vi "PostImagesONE_GRAPH_WORKING_PRE_LOOPIFY.vi"(6 "URL":string, 7 "Experiment Identifier":string, 8 "Transconductance..":refnum<vi>, 9 "Transconductance":refnum<vi>, 10 "Conductance..":refnum<vi>, 11 "Conductance":refnum<vi>) -> ()   [LabVIEW 2016]
uses:
  <vilib>/httpClient/MultipartData.ctl
  <vilib>/httpClient/POSTFile.vi
  <vilib>/httpClient/LabVIEWHTTPClient.lvlib
panel:
  out "error out 4":errorcluster
  out "error out 3":errorcluster
  out "error out 2":errorcluster
  out "error out":errorcluster
  out "appended path 4":path
  out "appended path 3":path
  out "appended path 2":path
  out "appended path":path
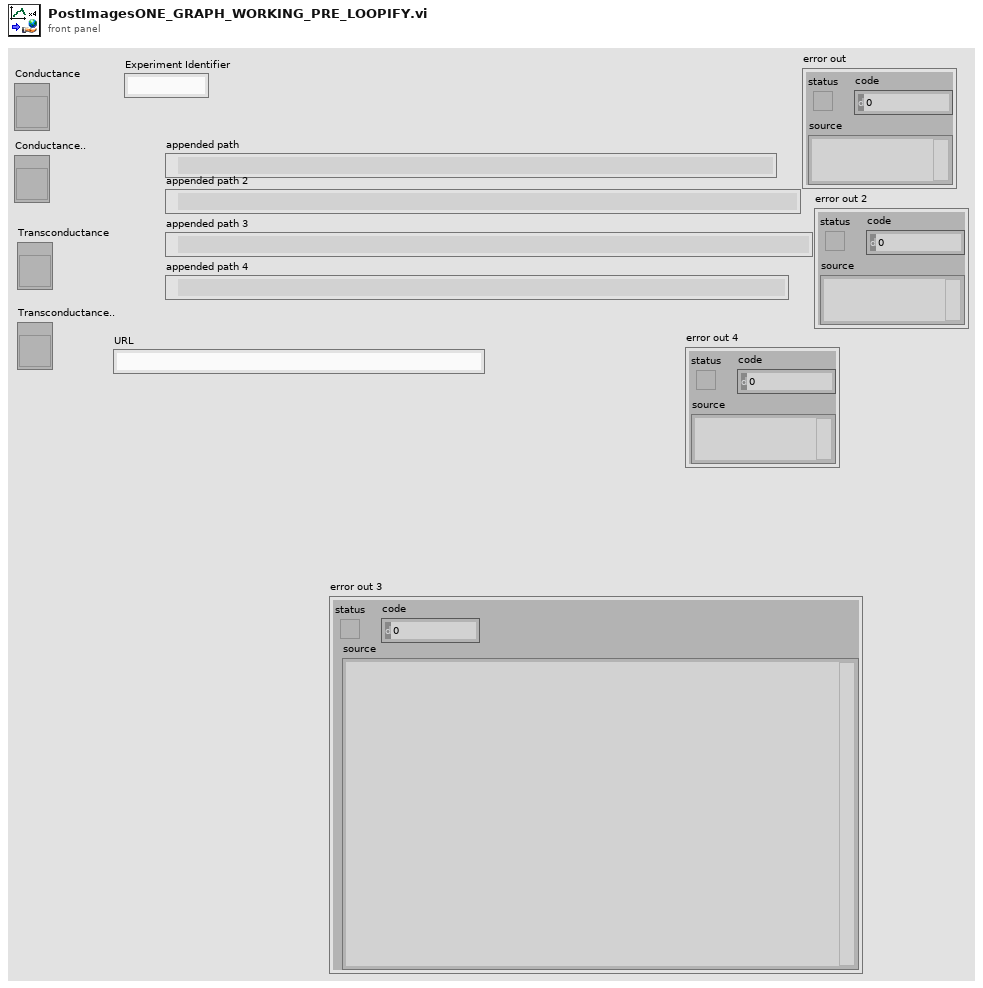
[diagram p1: front panel]
types:
  T1 = typedef "LabVIEWHTTPClient.lvlib/MultipartData.ctl" = cluster{"Name":string, "Value":string, "File":path, "Filename":string, "MIME type":string}
  T2 = typedef "imagedata.ctl" = cluster{"image type":i32, "image depth":i32, "image":u8[], "mask":u8[], "colors":u32[], "Rectangle":cluster{"left":i16, "top":i16, "right":i16, "bottom":i16}}
  T3 = typedef "LabVIEWHTTPClient.lvlib/ClientHandle.ctl" = refnum<k1>
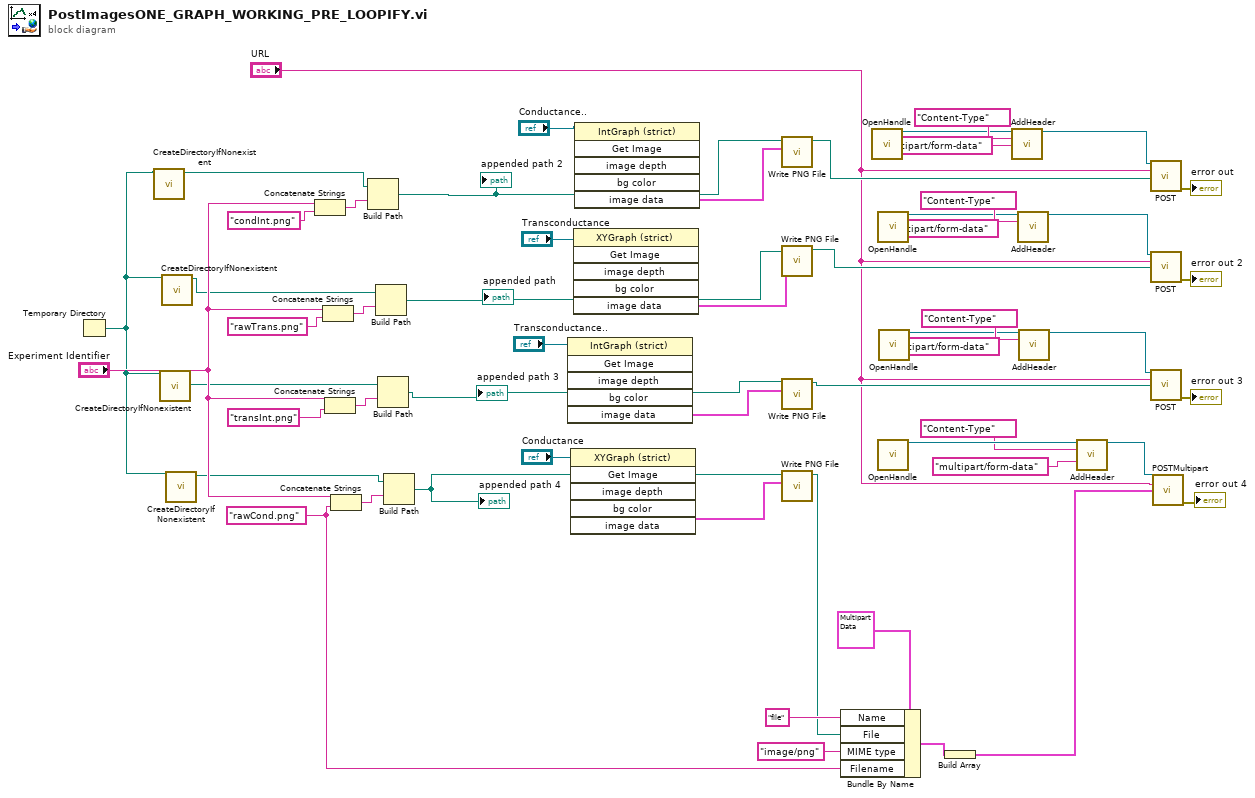
[diagram p0: block diagram]
diagram:
  (unwired) "multipart/form-data" ("value")
  (unwired) "multipart/form-data" ("value")
  w2 = "rawCond.png" ("name or relative path")
  n1 = Temporary Directory() -> (w29:path)
  n2 = call "CreateDirectoryIfNonexistent.vi"("selected path"=w29) -> ("path"=w33:path)  [unwired: 10 in]
  n3 = call "CreateDirectoryIfNonexistent.vi"("selected path"=w29) -> ("path"=w30:path)  [unwired: 10 in]
  n4 = call "CreateDirectoryIfNonexistent.vi"("selected path"=w29) -> ("path"=w32:path)  [unwired: 10 in]
  n5 = call "CreateDirectoryIfNonexistent.vi"("selected path"=w29) -> ("path"=w31:path)  [unwired: 10 in]
  n6 = Concatenate Strings("Experiment Identifier", "condInt.png" ("name or relative path")) -> (w43:string)
  n7 = Concatenate Strings("Experiment Identifier", "rawTrans.png" ("name or relative path")) -> (w42:string)
  n8 = Concatenate Strings("Experiment Identifier", "transInt.png" ("name or relative path")) -> (w41:string)
  n9 = Concatenate Strings("Experiment Identifier", w2) -> (w10:string)
  n10 = Build Path(base path=w33, name or relative path=w43) -> (appended path=w37:path)
  "appended path 2" <- w37
  n11 = Build Path(base path=w32, name or relative path=w42) -> (appended path=w36:path)
  "appended path" <- w36
  n12 = Build Path(base path=w30, name or relative path=w41) -> (appended path=w35:path)
  "appended path 3" <- w35
  n13 = Build Path(base path=w31, name or relative path=w10) -> (appended path=w34:path)
  "appended path 4" <- w34
  n14 = invoke class="IntGraph (strict)" method="Get Image"(reference="Transconductance..") -> ("image data"=w52:T2)  [unwired: 5 in, 5 out]
  n15 = invoke class="XYGraph (strict)" method="Get Image"(reference="Conductance") -> ("image data"=w50:T2)  [unwired: 5 in, 5 out]
  n16 = invoke class="XYGraph (strict)" method="Get Image"(reference="Transconductance") -> ("image data"=w49:T2)  [unwired: 5 in, 5 out]
  n17 = invoke class="IntGraph (strict)" method="Get Image"(reference="Conductance..") -> ("image data"=w54:T2)  [unwired: 5 in, 5 out]
  n18 = call <vilib>:"Write PNG File.vi"("image data"=w54, "path to PNG file"=w37) -> ("path"=w13:path)  [unwired: 8 in, 1 out]
  n19 = call <vilib>:"Write PNG File.vi"("image data"=w49, "path to PNG file"=w36) -> ("path"=w46:path)  [unwired: 8 in, 1 out]
  n20 = call <vilib>:"Write PNG File.vi"("image data"=w52, "path to PNG file"=w35) -> ("path"=w45:path)  [unwired: 8 in, 1 out]
  n21 = call <vilib>:"Write PNG File.vi"("image data"=w50, "path to PNG file"=w34) -> ("path"=w6:path)  [unwired: 8 in, 1 out]
  n22 = Bundle By Name(cluster=T1 {"Name"="", "Value"="", "File"=path "", "Filename"="", "MIME type"="application/octet-stream"} ("Element"), "Name"="file", "File"=w6, "MIME type"="image/png", "Filename"=w2) -> (w9:T1)
  n23 = call <vilib>:"OpenHandle.vi"() -> ("client handle out"=w23:T3)  [unwired: 14 in, 1 out]
  n24 = call <vilib>:"OpenHandle.vi"() -> ("client handle out"=w21:T3)  [unwired: 14 in, 1 out]
  n25 = call <vilib>:"OpenHandle.vi"() -> ("client handle out"=w18:T3)  [unwired: 14 in, 1 out]
  n26 = call <vilib>:"OpenHandle.vi"() -> ("client handle out"=w19:T3)  [unwired: 14 in, 1 out]
  n27 = Build Array(w9) -> (w8:T1[])
  n28 = call <vilib>:"AddHeader.vi"("client handle"=w23, "header"="Content-Type", "value"="multipart/form-data") -> ("client handle out"=w14:T3)  [unwired: 11 in, 1 out]
  n29 = call <vilib>:"AddHeader.vi"("client handle"=w21, "header"="Content-Type") -> ("client handle out"=w16:T3)  [unwired: 12 in, 1 out]
  n30 = call <vilib>:"AddHeader.vi"("client handle"=w19, "header"="Content-Type") -> ("client handle out"=w15:T3)  [unwired: 12 in, 1 out]
  n31 = call <vilib>:"AddHeader.vi"("client handle"=w18, "header"="Content-Type", "value"="multipart/form-data") -> ("client handle out"=w12:T3)  [unwired: 11 in, 1 out]
  n32 = call-poly <vilib>:"POST.vi"("client handle"=w14, "url"="URL", "file"=w13) -> ("error out"=→"error out":errorcluster)  [unwired: 9 in, 3 out]
  n33 = call-poly <vilib>:"POST.vi"("client handle"=w16, "url"="URL", "file"=w46) -> ("error out"=→"error out 2":errorcluster)  [unwired: 9 in, 3 out]
  n34 = call-poly <vilib>:"POST.vi"("client handle"=w15, "url"="URL", "file"=w45) -> ("error out"=→"error out 3":errorcluster)  [unwired: 9 in, 3 out]
  n35 = call <vilib>:"POSTMultipart.vi"("client handle"=w12, "url"="URL", "data"=w8) -> ("error out"=→"error out 4":errorcluster)  [unwired: 9 in, 3 out]
